vi "GetTeamListings.vi"() -> ()   [LabVIEW 2014, in "FIRST Events API.lvlib"]
uses:
  FIRST Events API.lvlib
  Event Alliances.ctl
  FRC Events.ctl
panel:
  out "value":T1
  out "error out":errorcluster
  out "body":string
  out "headers":string
  out "Generated URL":string
  in  "Append to URL":string
  # "This VI does not work right now, and I do not know why."
  # "This will be replaced later."
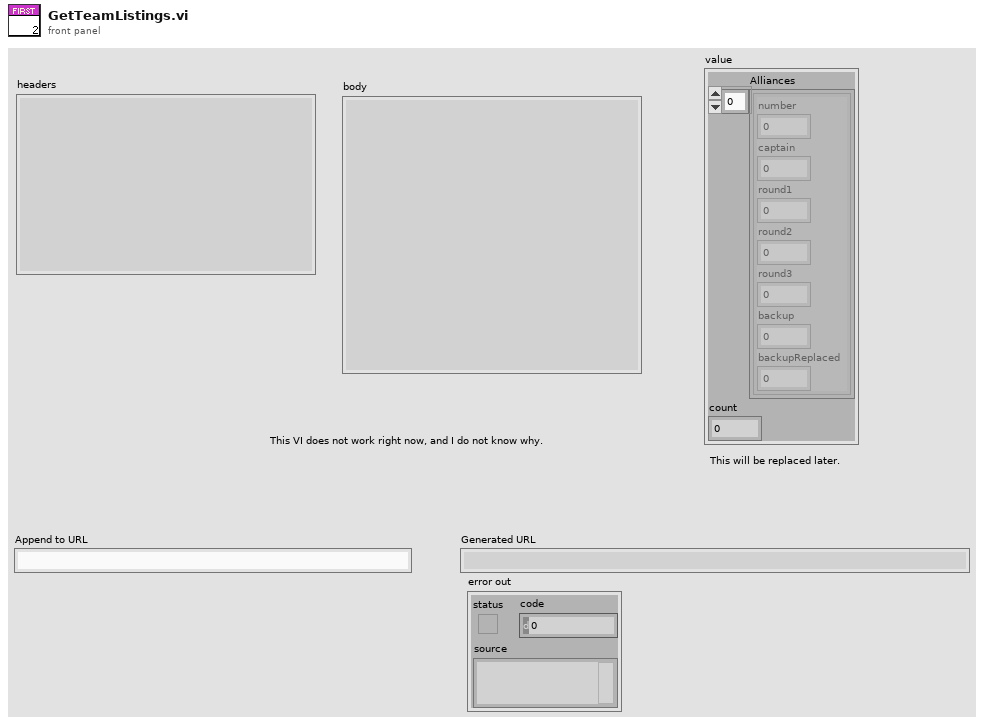
[diagram p1: front panel]
types:
  T1 = typedef "FIRST Events API.lvlib/Event Alliances.ctl" = cluster{"Alliances":cluster{"number":i32, "captain":i32, "round1":i32, "round2":i32, "round3":i32, "backup":i32, "backupReplaced":i32}[], "count":i32}
  T2 = typedef "FIRST Events API.lvlib/FRC Events.ctl" = enum16{"GetEventAllianceSelection", "Ancillary", "GetTeamListings"}
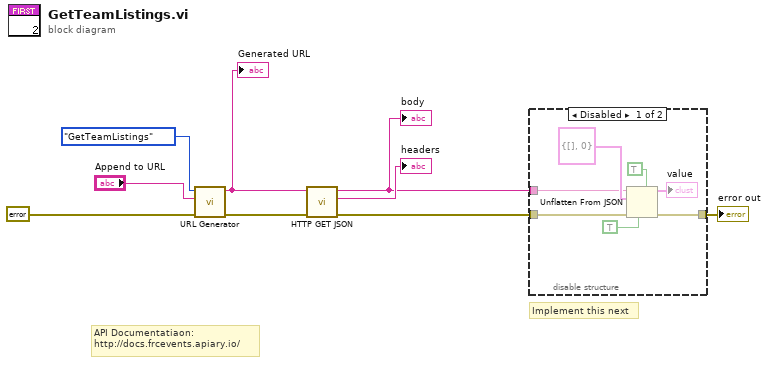
[diagram p0: block diagram]
diagram:
  # "Implement this next"
  # "API Documentatiaon:\nhttp://docs.frcevents.apiary.io/"
  n1 = call "URL Generator.vi"("error in (no error)"=errorcluster {"status"=FALSE, "code"=0, "source"=""}, "Append URL"="Append to URL", "API Command"=FRC_Events."GetTeamListings") -> ("error out"=w4:errorcluster, "Generated URL"=w7:string)  [unwired: 7 in]
  "Generated URL" <- w7
  n2 = call "HTTP GET JSON.vi"("error in (no error)"=w4, "Generated URL"=w7) -> ("error out"=w2:errorcluster, "headers"=→"headers":string, "body"=w3:string)  [unwired: 7 in]
  "body" <- w3
  n3 = disable-structure shown="Disabled" {
    disable-tunnel: w3 -> [w15 _]
    disable-tunnel: w2 -> [w14 _]
    disable-tunnel: [w13 _] -> w1
    frame Disabled {
      n4 = Unflatten From JSON(enable LabVIEW extensions? (T)=TRUE, JSON string=w15, type and defaults=T1 {"Alliances"=[], "count"=0} ("Event Alliances"), default null elements? (F)=TRUE, error in (no error)=w14) -> (value=→"value":T1, error out=w13:errorcluster)  [unwired: 2 in]
    }
    frame Enabled {
    }
  }
  "error out" <- w1
